vi "例6-14.vi"() -> ()   [LabVIEW 2019]
uses:
  <vilib>/Analysis/4window.llb/windowTd.ctl
  <vilib>/measure/macond.llb/IIR Filter for 1 Chan.vi
  <vilib>/measure/maspectr.llb/Frequency Response Function (Mag-Phase) 1-1.vi
  <vilib>/measure/NI_MABase.lvlib
  <vilib>/measure/NI_MAPro.lvlib
  <vilib>/Analysis/NI_AALPro.lvlib
panel:
  out "频率响应":cluster{"f0":dbl, "df":dbl, "magnitude":dbl[]}(graph)
  in  "高截止频率":dbl=3800.0
  in  "低截止频率":dbl=2000.0
  in  "阶数":dbl=6.0
  # "IIR滤波器规范"
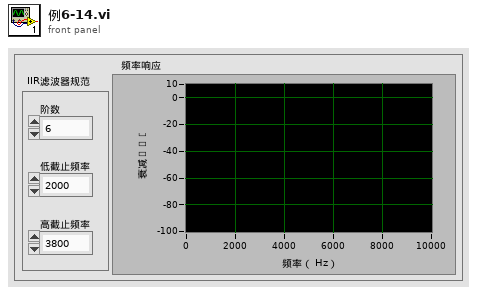
[diagram p1: front panel]
types:
  T1 = enum16{"No averaging", "Vector averaging", "RMS averaging", "Peak hold"}
  T2 = cluster{"averaging mode":enum16{"No averaging", "Vector averaging", "RMS averaging", "Peak hold"}, "weighting mode":enum16{"Linear", "Exponential"}, "number of averages":u32}
  T3 = cluster{"dB On (F)":bool, "unwrap phase (F)":bool, "convert to degree (F)":bool}
  T4 = typedef "NI_AALPro.lvlib/windowTd.ctl" = u32
  T5 = cluster{"Topology":enum16{"Off", "Butterworth", "Chebyshev", "Inverse Chebyshev", "Elliptic", "Bessel"}, "Type":enum16{"Lowpass", "Highpass", "Bandpass", "Bandstop"}, "Order":i32, "Lower Fc":dbl, "Upper Fc":dbl, "PB Ripple":dbl, "SB Attenuation":dbl}
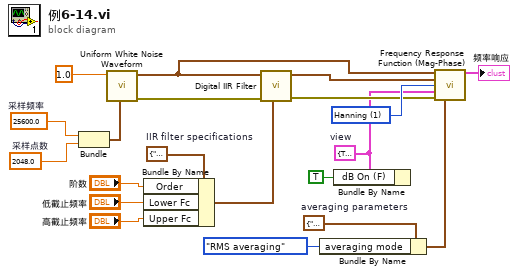
[diagram p0: block diagram]
diagram:
  w5 = T2 {"averaging mode"=enum."RMS averaging", "weighting mode"=enum."Exponential", "number of averages"=10}  # averaging parameters
  w3 = T3 {"dB On (F)"=TRUE, "unwrap phase (F)"=FALSE, "convert to degree (F)"=FALSE}  # view
  w13 = T4 1 items=["矩形"=0, "Hanning"=1, "Hamming"=2, "Blackman-Harris"=3, "Exact Blackman"=4, "Blackman"=5, "Flat Top"=6, "4阶Blackman-Harris "=7, "7阶Blackman-Harris"=8, "Low Sidelobe"=9, "Blackman Nuttall"=11, "三角"=30, "Bartlett-Hanning"=31, "Bohman"=32, "Parzen"=33, "Welch"=34, "Kaiser"=60, "Dolph-Chebyshev"=61, "高斯"=62] ("window")
  w2 = T5 {"Topology"=enum."Butterworth", "Type"=enum."Bandpass", "Order"=7, "Lower Fc"=2000.0, "Upper Fc"=3800.0, "PB Ripple"=0.025, "SB Attenuation"=90.0}  # IIR filter specifications
  w19 = 2048.0  # 采样点数
  w20 = 25600.0  # 采样频率
  n1 = Bundle("采样频率"=w20, "采样点数"=w19) -> (w18:cluster{" 采样频率":dbl, "采样点数":dbl})  [unwired: 1 in]
  n2 = call <vilib>:"Uniform White Noise Waveform.vi"("sampling info"=w18, "amplitude"=1.0) -> ("error out"=w16:errorcluster, "signal out"=w15:waveform(dbl))  [unwired: 8 in]
  n3 = Bundle By Name(cluster=w2, "Order"="阶数", "Lower Fc"="低截止频率", "Upper Fc"="高截止频率") -> (w8:T5)
  n4 = call-poly <vilib>:"Digital IIR Filter.vi"("IIR filter specifications"=w8, "error in (no error)"=w16, "signal in"=w15) -> ("error out"=w7:errorcluster, "signal out"=w14:waveform(dbl))  [unwired: 6 in, 1 out]
  n5 = Bundle By Name(cluster=w5, "averaging mode"=T1."RMS averaging") -> (w1:T2)
  n6 = Bundle By Name(cluster=w3, "dB On (F)"=TRUE) -> ()  [unwired: 1 out]
  n7 = call-poly <vilib>:"Frequency Response Function (Mag-Phase).vi"("time signal X"=w15, "time signal Y"=w14, "window"=w13, "view"=w3, "error in (no error)"=w7, "averaging parameters"=w1) -> ("magnitude"=→"频率响应":cluster{"f0":dbl, "df":dbl, "magnitude":dbl[]})  [unwired: 4 in, 5 out]
